vi "EinfacheRegelung.vi"() -> ()   [LabVIEW 2019]
panel:
  in  "Abkühlung+Vacuum":bool
  in  "Temperatur Regelung":bool
  in  "Timer (Stunde)":dbl
  out "Cold Plate":dbl(graph)
  out "Sample Plate":dbl(graph)
  out "Cold Plate Temperature":dbl
  in  "Stopp":bool
  in  "Sample":dbl
  in  "Cold Plate":dbl
  out "Sample Temperature":dbl
  out "AttoDryCode":path
  out "Status":dbl
  # "Während des Tests"
  # "Input"
  # "Bedingungen"
  # "OFF"
  # "ON"
  # "OFF"
  # "ON"
  # "Ensure the chamber is sealed properly"
  # "Temperaturen"
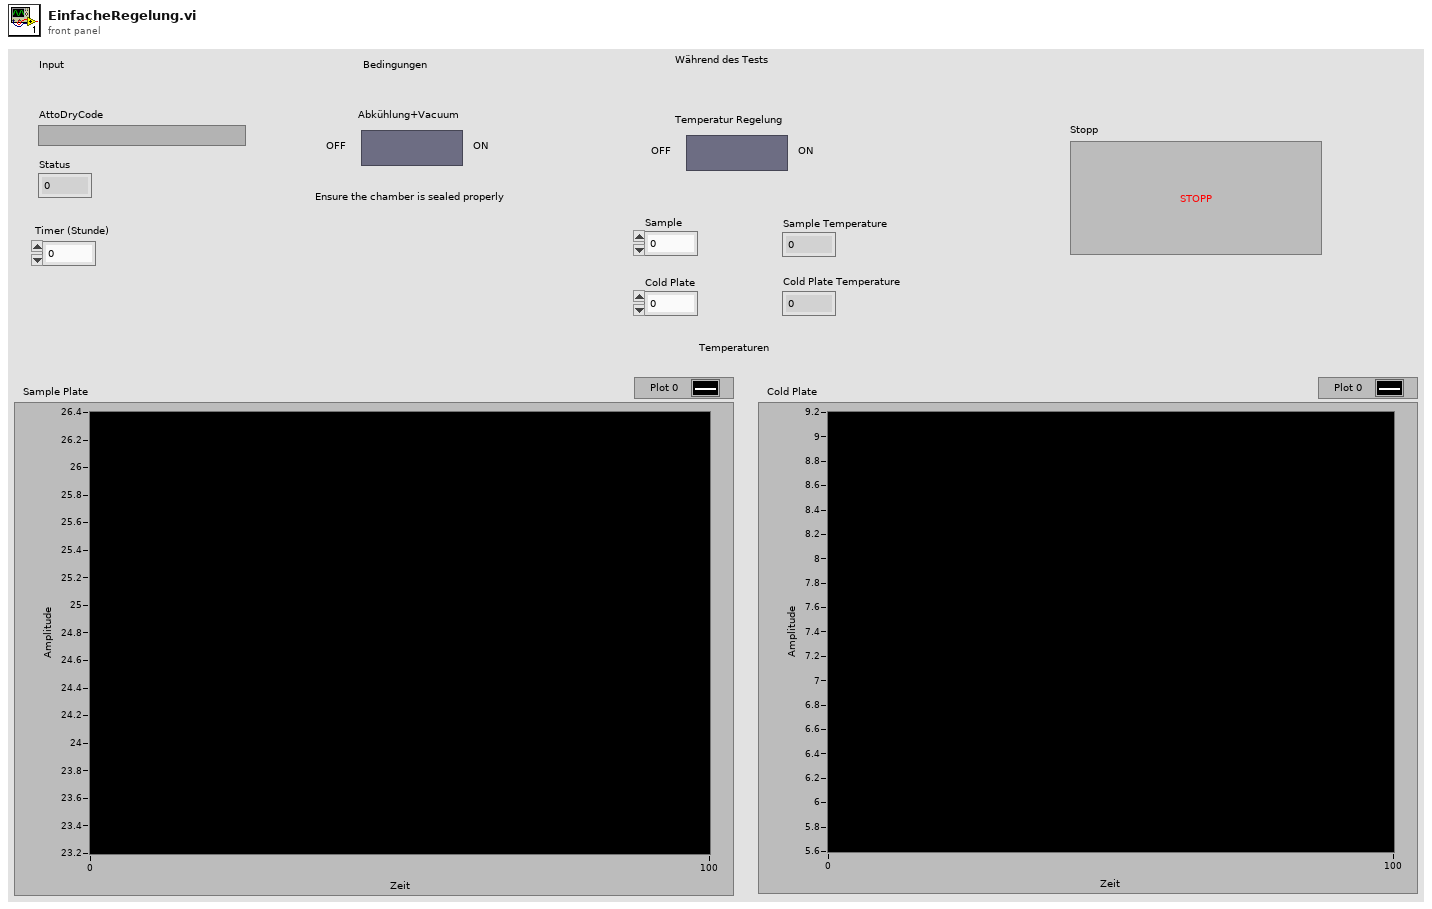
[diagram p1: front panel]
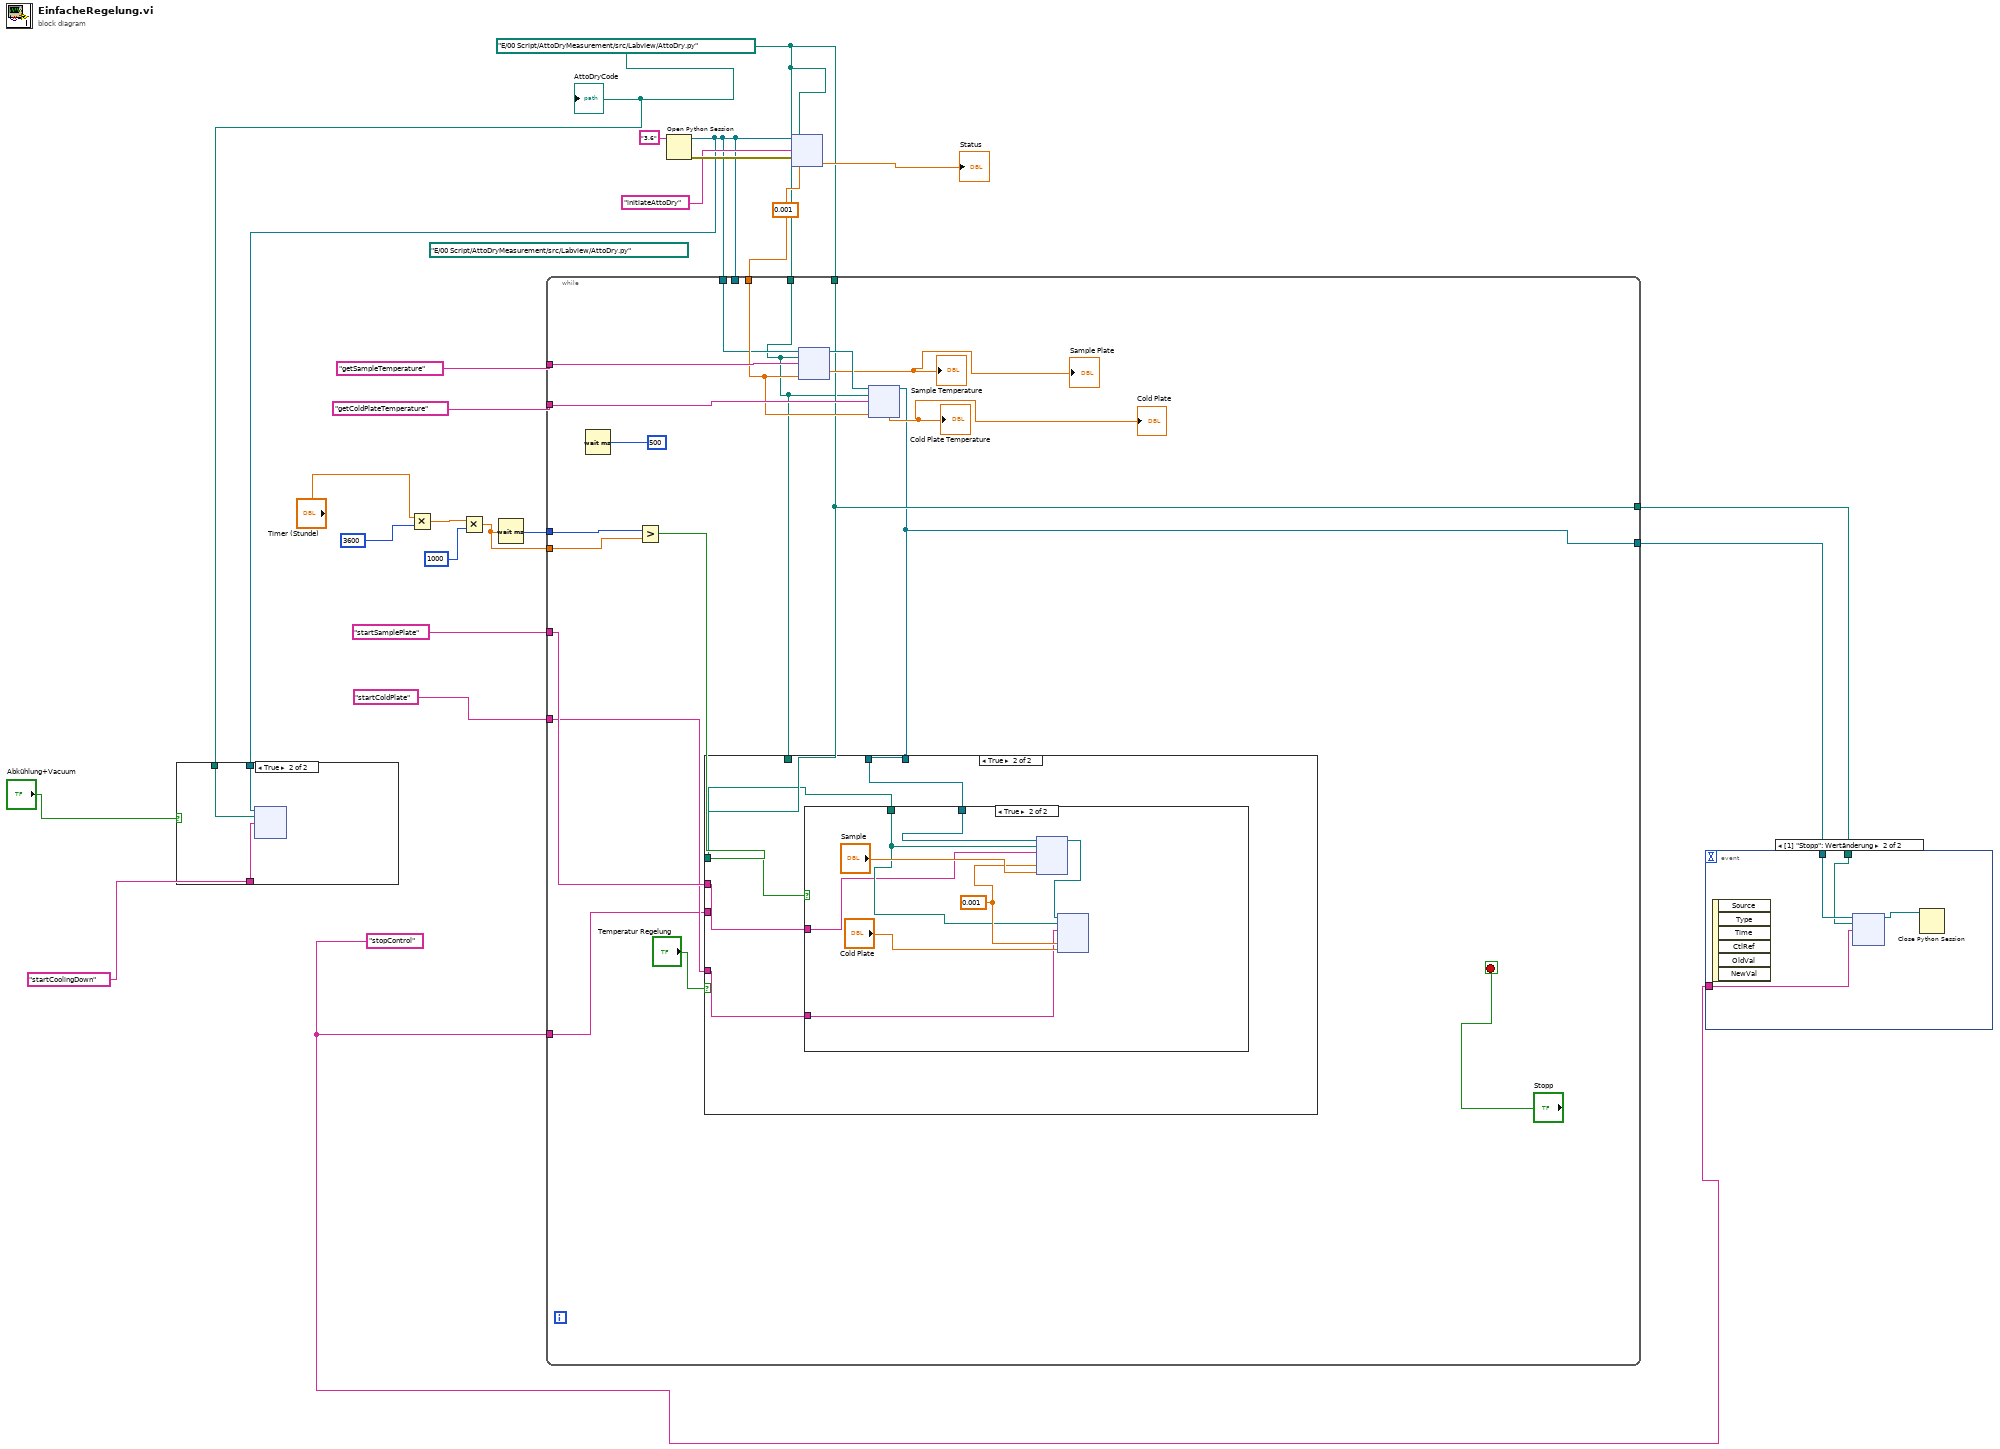
[diagram p0: block diagram]
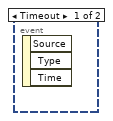
[diagram p3: hidden frame]
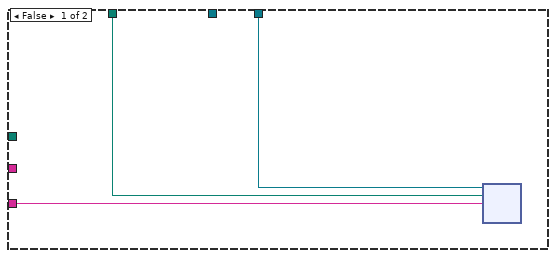
[diagram p4: hidden frame]
diagram:
  w5 = "stopControl" ("Funktionsname")
  w17 = 0.001
  (unwired) path "E:/00 Script/AttoDryMeasurement/src/Labview/AttoDry.py" ("Pfad")
  w1 = path "E:/00 Script/AttoDryMeasurement/src/Labview/AttoDry.py" ("Pfad")
  n1 = Multiply(x="Timer (Stunde)", y=u32 3600 ("Zu wartende ms")) -> (x*y=w13:dbl)
  n2 = Multiply(x=w13, y=u32 1000 ("Zu wartende ms")) -> (x*y=w11:dbl)
  n3 = Wait (ms)(milliseconds to wait=w11) -> (millisecond timer value=w15:u32)
  n4 = Open Python Session(python version="3.6" ("Python-Version")) -> (session out=w2:refnum<k35>, error out=w22:errorcluster)  [unwired: 2 in]
  n5 = case shown="True" "Abkühlung+Vacuum" {
    tunnel: "startCoolingDown" ("Funktionsname") -> [_ w25]
    tunnel: w2 -> [_ w24]
    tunnel: w1 -> [_ w23]
    frame False {
    }
    frame True {
      n6 = node(w24, w23, w25) -> ()  [unwired: 3 in, 4 out]
    }
  }
  n7 = while {
    tunnel: w2 -> [w34]
    tunnel: w1 -> [w27]
    tunnel: "getSampleTemperature" ("Funktionsname") -> [w44]
    tunnel: w17 -> [w39]
    tunnel: "getColdPlateTemperature" ("Funktionsname") -> [w40]
    tunnel: w15 -> [w36]
    tunnel: w11 -> [w35]
    tunnel: w1 -> [w31]
    tunnel: w2 -> [_]
    tunnel: [w26] -> w6
    tunnel: "startSamplePlate" ("Funktionsname") -> [w30]
    tunnel: "startColdPlate" ("Funktionsname") -> [w29]
    tunnel: [w31] -> w7
    tunnel: w5 -> [w28]
    stop <- "Stopp" stop-if-true
    n8 = Wait (ms)(milliseconds to wait=u32 500 ("Zu wartende ms")) -> ()  [unwired: 1 out]
    n9 = Greater?(x=w36, y=w35) -> (0:w32:bool)
    n10 = node(w34, w27, w44, w39) -> (w41:refnum<k35>, →"Sample Temperature" →"Sample Plate":dbl)  [unwired: 1 in, 3 out]
    n11 = node(w41, w27, w40, w39) -> (w26:refnum<k35>, →"Cold Plate Temperature" →"Cold Plate":dbl)  [unwired: 1 in, 3 out]
    n12 = case shown="True" "Temperatur Regelung" {
      tunnel: w32 -> [_ w52]
      tunnel: w26 -> [_ w51]
      tunnel: w31 -> [_ w50]
      tunnel: w30 -> [_ w49]
      tunnel: w29 -> [_ w48]
      tunnel: w28 -> [w47 _]
      tunnel: w27 -> [w46 _]
      tunnel: w26 -> [w45 _]
      frame False {
        n13 = node(w45, w46, w47) -> ()  [unwired: 3 in, 4 out]
      }
      frame True {
        n14 = case shown="True" w52 {
          tunnel: w51 -> [_ w57]
          tunnel: w50 -> [_ w56]
          tunnel: w49 -> [_ w54]
          tunnel: w48 -> [_ w53]
          frame False {
          }
          frame True {
            w59 = 0.001
            n15 = node(w57, w56, w54, w59, "Sample") -> (w55:refnum<k35>)  [unwired: 3 in, 3 out]
            n16 = node(w55, w56, w53, w59, "Cold Plate") -> ()  [unwired: 3 in, 4 out]
          }
        }
      }
    }
  }
  n17 = node(w2, w1, "initiateAttoDry" ("Funktionsname"), w22, w17) -> (→"Status":dbl)  [unwired: 4 out]
  n18 = event shown="[1] \"Stopp\": Wertänderung" {
    selector: _ -> [_ _]
    dyn-events: _ -> [_ _]
    timeout: _ -> [_ _]
    tunnel: w5 -> [_ w64]
    tunnel: w7 -> [_ w62]
    tunnel: w6 -> [_ w63]
    event Timeout {
      n19 = event-data() -> ()  [unwired: 1 in, 3 out]
    }
    event "Stopp": Value Change {
      n20 = event-data() -> ()  [unwired: 1 in, 6 out]
      n21 = node(w63, w62, w64) -> (w61:refnum<k35>)  [unwired: 3 in, 3 out]
      n22 = Close Python Session(session in=w61) -> ()  [unwired: 1 in, 1 out]
    }
  }
  "AttoDryCode" <- w1
